vi "PXI-Read DI Buffers.vi"(0 "DI Tasks":T1[](array[typedef]), 1 "Samples to skip":i32, 7 "Samples per channel":i32, 11 "error in (no error)":errorcluster, 12 "timeout (sec)":dbl=10.0 format="%0.2f") -> (8 "DI Waveforms":bool[][](array[boolean]), 15 "error out":errorcluster)   [LabVIEW 2020]
uses:
  Type Defs/Task Struct.ctl
  <vilib>/DAQmx/read.llb/DAQmx Read (Digital Wfm 1Chan NSamp).vi
  <vilib>/DAQmx/miscellaneous.llb/DAQmx Fill In Error Info.vi
  <vilib>/Waveform/DWDTOps.llb/DWDT Digital to Boolean Array.vi
panel:
  out "Digital Waveform Graph":digitalwaveform(graph)
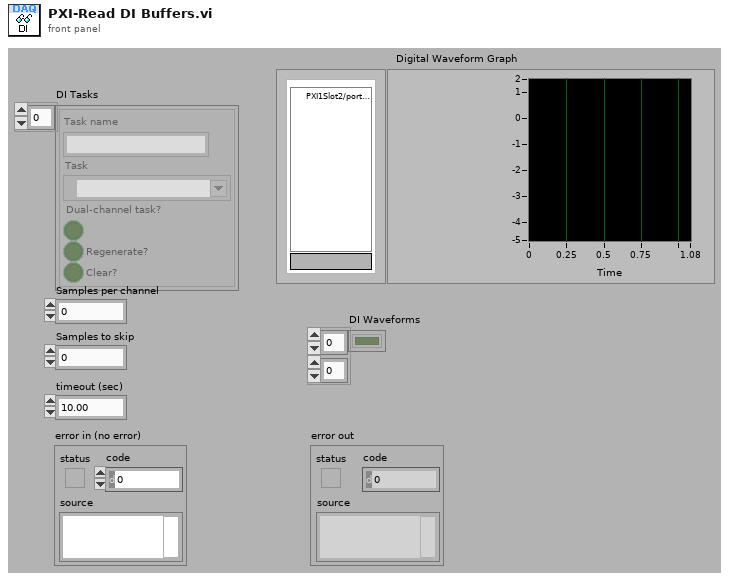
[diagram p1: front panel]
types:
  T1 = typedef "Task Struct.ctl" = cluster{"Task name":string, "Task":refnum<k21>, "Dual-channel task?":bool, "Regenerate?":bool, "Clear?":bool}
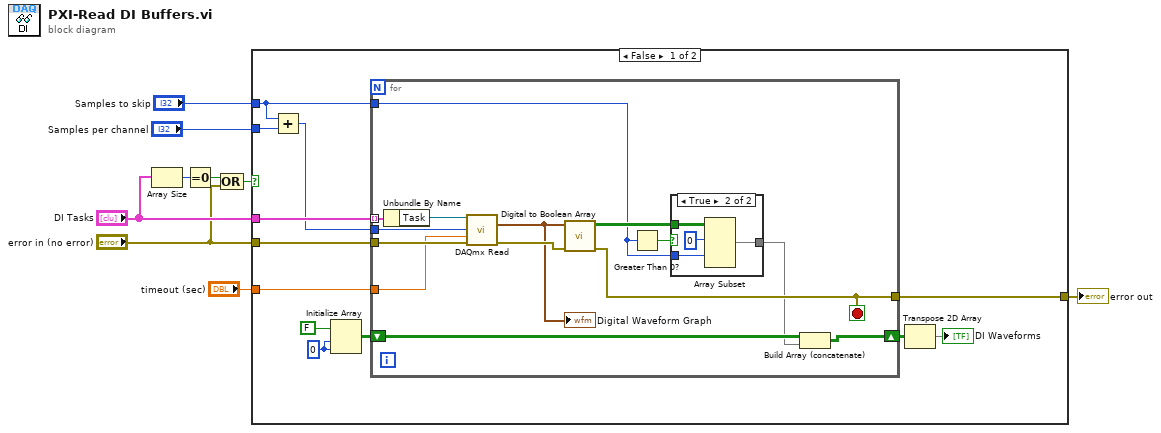
[diagram p0: block diagram]
diagram:
  n1 = Array Size(array="DI Tasks") -> (size(s)=w8:i32)
  n2 = Equal To 0?(x=w8) -> (x = 0?=w7:bool)
  n3 = Compound Arithmetic op=OR(w7, "error in (no error)") -> (w5:bool)
  n4 = case shown="False" w5 {
    tunnel: "error in (no error)" -> [w21 w41]
    tunnel: [w20 w41] -> w9
    tunnel: "DI Tasks" -> [w19 _]
    tunnel: "timeout (sec)" -> [w14 _]
    tunnel: "Samples per channel" -> [w12 _]
    tunnel: "Samples to skip" -> [w10 _]
    frame False {
      w17 = 0 ("dimension size")
      n5 = Add(x=w10, y=w12) -> (x+y=w11:i32)
      n6 = Initialize Array(FALSE, w17, w17) -> (w16:bool[][])
      n7 = for {
        tunnel: w19 -> [w35] mode=indexing
        shift-right: [w32] -> w18
        shift-left: w16 -> [w33]
        tunnel: w21 -> [w34]
        tunnel: [w26] -> w20
        tunnel: w14 -> [w28]
        tunnel: w11 -> [w27]
        tunnel: w10 -> [w23]
        stop <- w26 stop-if-true
        n8 = Unbundle By Name(w35) -> ("Task"=w31:refnum<k21>)
        n9 = call-poly <vilib>:"DAQmx Read.vi"("task/channels in"=w31, "number of samples per channel"=w27, "timeout"=w28, "error in"=w34) -> ("data"=w29:digitalwaveform, "error out"=w30:errorcluster)  [unwired: 9 in, 1 out]
        "Digital Waveform Graph" <- w29
        n10 = call-poly <vilib>:"Digital to Boolean Array.vi"("error in (no error)"=w30, "digital waveform"=w29) -> ("error out"=w26:errorcluster, "boolean array"=w25:bool[][])  [unwired: 8 in]
        n11 = Greater Than 0?(x=w23) -> (x > 0?=w22:bool)
        n12 = case shown="True" w22 {
          tunnel: w25 -> [w36 w39]
          tunnel: [w36 w38] -> w24
          tunnel: w23 -> [_ w37]
          frame False {
          }
          frame True {
            n13 = Array Subset(array=w39, index (row)=0, index (col)=w37) -> (w38:bool[][])  [unwired: 2 in]
          }
        }
        n14 = Build Array (concatenate)(w33, w24) -> (w32:bool[][])
      }
      n15 = Transpose 2D Array(2D array=w18) -> (transposed array=→"DI Waveforms":bool[][])
    }
    frame True {
    }
  }
  "error out" <- w9
